vi "Button Toggle.vi"(11 "Button In":bool) -> (0 "One-Shot Out":bool, 3 "Toggle Out":bool)   [LabVIEW 2017]
doc: "The Button Toggle function basically converts a momentary action pushbutton input into a toggle type switch. It provides two outputs - \"Toggle\" which changes boolean state when the input pushbutton is pushed by the operator and \"One-Shot\" which provides a single pulsed True output when the button is pushed."
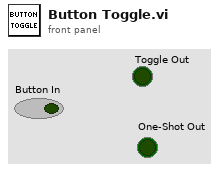
[diagram p1: front panel]
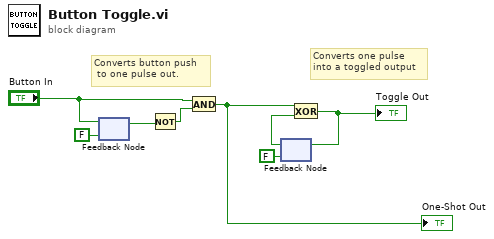
[diagram p0: block diagram]
diagram:
  # "Converts one pulse\ninto a toggled output"
  # "Converts button push\n to one pulse out."
  n1 = feedback #1(FALSE ("Button 1")) -> (w4:bool)
  n2 = feedback-in #1("Button In") -> ()
  n3 = Not(x=w4) -> (.not. x?=w5:bool)
  n4 = And(x="Button In", y=w5) -> (x .and. y?=w1:bool)
  "One-Shot Out" <- w1
  n5 = feedback #2(FALSE) -> (w2:bool)
  n6 = Exclusive Or(1:w2, 2:w1) -> (0:w3:bool)
  "Toggle Out" <- w3
  n7 = feedback-in #2(w3) -> ()
